vi "Main Data Log.vi"(8 "error in (no error)":errorcluster, 11 "main ref":T1) -> (0 "error out":errorcluster)   [LabVIEW 2025]
uses:
  controls/LAB-IQ UI Data.ctl
  <vilib>/Utility/file.llb/Write Delimited Spreadsheet (DBL).vi
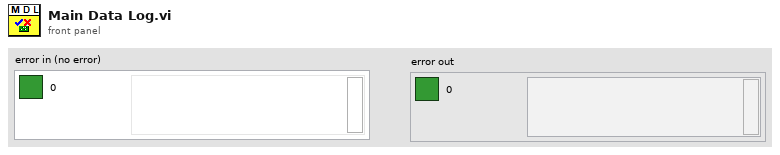
[diagram p1: front panel]
types:
  T1 = typedef "LAB-IQ UI Data.ctl" = cluster{"Main Home Screen":cluster{"GUI":refnum<vi>, "Platform Settings":refnum<vi>, "Configure":refnum<vi>, "Home":refnum<vi>, "EXIT":refnum<vi>, "service 2":refnum<vi>, "MainPage":refnum<vi>, "Analysis":refnum<vi>}, "Platform Settings":cluster{"mm/s  Surge":refnum<vi>, "Update Surge Speed":refnum<vi>, "Drive Error":refnum<vi>, "Disable Axis Jog Soft Limits":refnum<vi>, "mm/s  Sway":refnum<vi>, "Sway and Surge COM Status":refnum<vi>, "Heave COM Status":refnum<vi>, "Enable Platform":refnum<vi>, "Surge Forward Main":refnum<vi>, "Sway Right Main":refnum<vi>, "Sway Left Main":refnum<vi>, "Heave Down Main":refnum<vi>, "Heave Up main":refnum<vi>, "Update Sway Speed":refnum<vi>, "Update Heave Speed":refnum<vi>, "mm/s Heave":refnum<vi>, "mm/sec":refnum<vi>, "mm":refnum<vi>, "Surge Backward Main":refnum<vi>}, "Analysis Screen":cluster{"Analysis Home":refnum<vi>, "Surface Analysis":refnum<vi>, "Imaging":refnum<vi>, "Image Analysis":refnum<vi>, "Post Analysis":refnum<vi>}, "Config Screen":cluster{"Select Load Head":refnum<vi>, "Notes :":refnum<vi>, "FILE":refnum<vi>, "Sample ID :":refnum<vi>, "Operator ID :":refnum<vi>, "Operator Name :":refnum<vi>, "Auto":refnum<vi>}, "Motion Module":cluster{"zNL":refnum<vi>, "NL disp":refnum<vi>, "Rotary Tab":refnum<vi>, "Motion Direction:  3":refnum<vi>, "E.Velocity 2":refnum<vi>, "e.v/ssr 2":refnum<vi>, "Enter Fixed E.Velocity 2":refnum<vi>, "Enter Final SRR 2":refnum<vi>, "Enter initial SRR 2":refnum<vi>, "Enter Fixed SRR 2":refnum<vi>, "Enter the Final E.Velocity (m/s) 2":refnum<vi>, "Enter initial E.Velocity (m/s) 2":refnum<vi>, "Final Speed (RPM) 3":refnum<vi>, "Initial Speed (RPM) 2":refnum<vi>, "Enter the Final Velocity (m/s) 3":refnum<vi>, "Enter initial Velocity (m/s)  3":refnum<vi>, "Ramp Up 2":refnum<vi>, "TEST SELECTION":refnum<vi>, "SPEED SELECTION : ":refnum<vi>, "Angular Oscillation Set":refnum<vi>, "Traction":refnum<vi>, "Step Speed":refnum<vi>, "StepTable For Load-Speed":refnum<vi>, "StepTable For Speed":refnum<vi>, "Surge Forward MM":refnum<vi>, "Surge Backward MM":refnum<vi>, "M3 Image":refnum<vi>, "String 39":refnum<vi>, "Sway Left MM":refnum<vi>, "Sway Right MM":refnum<vi>, "Disable Axis Jog Soft Limits":refnum<vi>, "mm":refnum<vi>, "Heave Down MM":refnum<vi>, "Heave Up MM":refnum<vi>, "Wear Track Diameter (mm)":refnum<vi>, "Set WTD":refnum<vi>, "HomeScratch":refnum<vi>, "HomeRot":refnum<vi>, "PlaceModule":refnum<vi>, "Enter the Angle (Deg)":refnum<vi>, "Enter the Frequency (Hz)":refnum<vi>, "Motion Mode:":refnum<vi>, "LR Sway":refnum<vi>, "Rot Hor":refnum<vi>, "Scratch":refnum<vi>, "LR Cam":refnum<vi>, "MMBack":refnum<vi>, "MMNext":refnum<vi>, "Rot Ver":refnum<vi>, "Rotary Module Selection":refnum<vi>, "calculate rotary":refnum<vi>, "SPEED SELECTION : rotary":refnum<vi>, "Import 2":refnum<vi>, "Save 2":refnum<vi>, "File Path :  2":refnum<vi>, "String 45":refnum<vi>, "StepTable For Speed 3":refnum<vi>, "Enter the Speed(mm/sec)":refnum<vi>, "Enter the Speed(RPM)":refnum<vi>, "Enter Scratch Speed (mm/s):":refnum<vi>, "SwaySpeed Set":refnum<vi>, "Scartch Offset":refnum<vi>, "Motion type:":refnum<vi>, "HomeScratch 2":refnum<vi>, "Enter Scratch length (mm):":refnum<vi>, "Wear Track Diameter":refnum<vi>, "Rotary Speed Exced":refnum<vi>, "Scratch Mode":refnum<vi>, "No of Scratch":refnum<vi>}, "Environmental control":cluster{"Humidity  Status  3":refnum<vi>, "Low Temp  Status  2":refnum<vi>, "TK4 status 2":refnum<vi>, "Stage Temperature":refnum<vi>, "Sample Temperature":refnum<vi>, "Humidity (Amb)":refnum<vi>, "Clear List":refnum<vi>, "Add to list":refnum<vi>, "Wear":refnum<vi>, "Vibration":refnum<vi>, "Humidity (Chamber)":refnum<vi>, "Temperature (Chamber)":refnum<vi>, "ECR ":refnum<vi>, "Temperature (Amb)":refnum<vi>, "Microphone":refnum<vi>, "Acoustic Emission 3":refnum<vi>, "SNext":refnum<vi>, "APBack":refnum<vi>, "Enter the Temperature (°C):":refnum<vi>, "Enter the Stage \nTemperature (°C):":refnum<vi>, "Enter the Humidity (%Rh):":refnum<vi>, "Low Temp":refnum<vi>, "High Temp":refnum<vi>, "Humidity":refnum<vi>, "Sensors Picked":refnum<vi>}, "About Screen":cluster{"Password":refnum<vi>, "Home Service":refnum<vi>, "Advanced Setting":refnum<vi>, "About Tab":refnum<vi>, "ECR Port:":refnum<vi>, "Ramp Port:":refnum<vi>, "Installation/Replacement completed":refnum<vi>, "Loahead":refnum<vi>, "Heave and Surge COM Port:":refnum<vi>, "Sway COM Port:":refnum<vi>, "Temp Modbus:":refnum<vi>, "Humidity Port:":refnum<vi>, "Edit Gain Constants":refnum<vi>, "Save Gain Constants":refnum<vi>}, "Main Screen":cluster{"Main Screen Tab":refnum<vi>, "Angle and Frequency":refnum<vi>, "Stroke (mm)":refnum<vi>, "Angle (Deg)":refnum<vi>, "Main Speed Tab":refnum<vi>, "MTM MOTOR DISPLAY":refnum<vi>, "Disc Speed (m/sec)":refnum<vi>, "Ball Speed (m/sec)":refnum<vi>, "Disc Speed (RPM)":refnum<vi>, "Ball Speed (RPM)":refnum<vi>, "SPEED TAB":refnum<vi>, "Speed (m/sec)":refnum<vi>, "Set Speed (m/sec)":refnum<vi>, "Speed (RPM)":refnum<vi>, "Set Speed":refnum<vi>, "Time Tab":refnum<vi>, "Time ( HH:MM:SS ) 2":refnum<vi>, "Test Duration":refnum<vi>, "Test Duration 4":refnum<vi>, "TEST CYCLE":refnum<vi>, "TOTAL CYCLES":refnum<vi>, "Set Load (N)":refnum<vi>, "Temp Tabs":refnum<vi>, "Heater":refnum<vi>, "TK4 status":refnum<vi>, "ChamberTemp":refnum<vi>, "SetTmp":refnum<vi>, "Controller  Status":refnum<vi>, "ChamberTemp 2":refnum<vi>, "SetTmp 2":refnum<vi>, "Controller  Status 2":refnum<vi>, "ChamberTemp 3":refnum<vi>, "SetTmp 3":refnum<vi>, "Cooling":refnum<vi>, "Load Communication":refnum<vi>, "Ambient \nTemperature":refnum<vi>, "HumCOMStatus":refnum<vi>, "Ambient\n Humidity":refnum<vi>, "Freq (Hz)":refnum<vi>, "Load En":refnum<vi>, "NLt":refnum<vi>, "zNL 2":refnum<vi>, "Humidity On":refnum<vi>, "humidity disp":refnum<vi>, "Set Humidity":refnum<vi>, "NL disp 2":refnum<vi>, "Humidity On 2":refnum<vi>, "humidity disp 2":refnum<vi>, "Set Humidity 2":refnum<vi>, "NL disp 3":refnum<vi>, "AppLoadSeq scratch":refnum<vi>, "Stop Scratch":refnum<vi>, "ClrLog":refnum<vi>, "Trip Log":refnum<vi>, "STOP":refnum<vi>, "Start Test":refnum<vi>, "Test status":refnum<vi>, "AR Led":refnum<vi>, "Data":refnum<vi>, "Health":refnum<vi>, "Sway COM Status":refnum<vi>, "Heave COM Status":refnum<vi>, "Grp Tab":refnum<vi>, "Sub Graph":refnum<vi>, "SD (mm)":refnum<vi>, "Siliding distance Reset Graph":refnum<vi>, "SDGp":refnum<vi>, "Humidity Reset Graph":refnum<vi>, "HumrGp":refnum<vi>, "Acoustic Emission (mV)":refnum<vi>, "Aqucostic Reset Graph":refnum<vi>, "gACQUOS":refnum<vi>, "ECR RESET":refnum<vi>, "ECR":refnum<vi>, "Temperature Reset":refnum<vi>, "Acoustic Emission (mV) 2":refnum<vi>, "Aqucostic Reset Graph 2":refnum<vi>, "gACQUOS 2":refnum<vi>, "ECR RESET 2":refnum<vi>, "ECR 2":refnum<vi>, "Temperature Reset 2":refnum<vi>, "Temperature (deg c)":refnum<vi>, "Speed Reset Graph":refnum<vi>, "Speed Tab":refnum<vi>, "MTM DISC  SPEED":refnum<vi>, "MTM BALL SPEED":refnum<vi>, "speed mm/sec":refnum<vi>, "Hymidity":refnum<vi>, "Humidity Disable trip":refnum<vi>, "CoF Trip  2":refnum<vi>, "Depth Trip":refnum<vi>, "Weart Deapth":refnum<vi>, "Depth Reset Graph":refnum<vi>, "Weart":refnum<vi>, "Depthz":refnum<vi>, "Depth (µm)":refnum<vi>, "WearGp":refnum<vi>, "NL Trip 2":refnum<vi>, "Load pid":refnum<vi>, "Load Disable Trip":refnum<vi>, "Load Reset Graph":refnum<vi>, "NL Display 4":refnum<vi>, "Main Chart 3":refnum<vi>, "BACK":refnum<vi>, "Depth Trip 2":refnum<vi>, "COF TRIP ":refnum<vi>, "Friction Force (N)":refnum<vi>, "FF Reset Graph":refnum<vi>, "FF Disable Trip":refnum<vi>, "FF TRIP":refnum<vi>, "COF Disable Trip":refnum<vi>, "COF Reset Graph":refnum<vi>, "Start Test Temp":refnum<vi>, "zFF":refnum<vi>, "Friction Force (N) Graph":refnum<vi>, "Coefficient of Friction":refnum<vi>, "Scratch Start Test":refnum<vi>, "FF Tab":refnum<vi>, "Cyclic Friction Force (N)":refnum<vi>, "CZ FF":refnum<vi>, "Cyclic Friction Force (N) Graph":refnum<vi>, "Cyclic Coefficient of Friction":refnum<vi>, "Cyclic FF TRIP":refnum<vi>, "Cyclic FF Disable Trip":refnum<vi>, "cyclic COF Disable Trip":refnum<vi>, "cyclic COF TRIP":refnum<vi>, "cyclic COF Reset Graph":refnum<vi>, "Cyclic FF Reset Graph":refnum<vi>, "Test Trip":refnum<vi>, "Multi Scratch Pass":refnum<vi>}, "Loading":cluster{"Indentation":refnum<vi>, "Reference Sample":refnum<vi>, "Load Cell Communication Slide":refnum<vi>, "com 3":refnum<vi>, "com":refnum<vi>, "DecaForce COM Status":refnum<vi>, "Update":refnum<vi>, "Clear 3":refnum<vi>, "seq":refnum<vi>, "Stribeck table":refnum<vi>, "Stribeck Table  For loading":refnum<vi>, "Loading Mode":refnum<vi>, "Enter the Final Load (N)":refnum<vi>, "Enter the CoF Trip":refnum<vi>, "Enter the Friction Force Trip":refnum<vi>, "Enter the Normal load Trip":refnum<vi>, "Enter the Load  (N)":refnum<vi>, "KiloForce":refnum<vi>, "DecaForce ":refnum<vi>, "MicroForce":refnum<vi>, "LHBack":refnum<vi>, "LHNext":refnum<vi>, "Enter the Loading Rate (N/min)":refnum<vi>, "Message":refnum<vi>, "Warning 2":refnum<vi>, "SSP 0.75":refnum<vi>, "SSP 0.5":refnum<vi>, "SSP 0.3":refnum<vi>, "Warning":refnum<vi>, "gui GIF":refnum<vi>, "Communication is established":refnum<vi>, "AppLoad 4":refnum<vi>, "Multipoint":refnum<vi>, "Load Selection":refnum<vi>}, "PID":cluster{"Ramp MulFac":refnum<vi>, "pulses LoadDiffRamp(2..10)":refnum<vi>, "PulseControlRamp(diff<=3N)":refnum<vi>, "SetLoadDeadband(%) Load(0-10N)":refnum<vi>, "PID gains out delay (microForce)":refnum<vi>, "Ramp":refnum<vi>, "Gain 2":refnum<vi>, "pulses LoadDiff(2..10)":refnum<vi>, "pulses LoadDiff(11..50)":refnum<vi>, "PulseControl(diff<=3N)":refnum<vi>, "SetLoadDeadband(%)  2":refnum<vi>, "Dummy Run":refnum<vi>, "Vertical load (N)":refnum<vi>, "AutoTune":refnum<vi>, "Offset 3 ":refnum<vi>, "apply load":refnum<vi>, "Offset  3":refnum<vi>, "apply load 2":refnum<vi>, "Enter ByPass Load":refnum<vi>, "reinit 3":refnum<vi>, "output range delay":refnum<vi>, "PID gains out delay":refnum<vi>, "Bypass Load":refnum<vi>, "pulsesSent":refnum<vi>, "pulses ":refnum<vi>, "actpid":refnum<vi>, "gFF Rot":refnum<vi>, "pulses LoadDiff(21..1000)":refnum<vi>, "Delay":refnum<vi>, "deadband":refnum<vi>}, "Config Parameters":cluster{"Tab Control 3":refnum<vi>, "Tab Control 19":refnum<vi>, "SAMPLES":refnum<vi>, "Re-initilaize":refnum<vi>, "Filter ON/OFF":refnum<vi>, "TracHomeSurgeOffsetCounts 10MM":refnum<vi>, "TracHomeSwayOffsetCounts 10MM":refnum<vi>, "Acoustic Emission:":refnum<vi>, "Apply Filter (FF)":refnum<vi>, "Filter% 2":refnum<vi>, "Apply Filter (Load)":refnum<vi>, "Filter% ":refnum<vi>, "Sway distance (mm)":refnum<vi>, "Surge distance (mm)":refnum<vi>, "DataSavingLoopDelay(ms)":refnum<vi>, "SAVE 2":refnum<vi>, "Enter Distance":refnum<vi>, "Sway Counts:":refnum<vi>, "Distance (mm): 3":refnum<vi>, "Surge Counts:":refnum<vi>, "Distance (mm): 2":refnum<vi>, "Distance (mm):":refnum<vi>, "Heave Counts:":refnum<vi>, "LRMHomeSurgeOffsetCounts":refnum<vi>, "LRMHomeSwayOffsetCounts":refnum<vi>, "TracHomeSurgeOffsetCounts 20MM":refnum<vi>, "TracHomeSwayOffsetCounts 20MM":refnum<vi>, "RotHomeSwayOffsetCounts":refnum<vi>, "RotHomeSurgeOffsetCounts":refnum<vi>, "Heave distance":refnum<vi>, "Zmm":refnum<vi>, "Heave Pulses/mm":refnum<vi>, "Surge Pulses/mm":refnum<vi>, "Sway Pulses/mm":refnum<vi>, "Heave Pitch":refnum<vi>, "Surge Pitch":refnum<vi>, "Sway Pitch":refnum<vi>, "Heave PPR":refnum<vi>, "Surge PPR":refnum<vi>, "Sway PPR":refnum<vi>, "Tab Control 5":refnum<vi>, "Tab Control 14":refnum<vi>, "Tab Control 26":refnum<vi>, "AE":refnum<vi>, "Heave Loop Delay":refnum<vi>, "Heave PID Speed":refnum<vi>, "Surge Jog Speed":refnum<vi>, "Heave Jog Speed":refnum<vi>, "Sway Loop Delay":refnum<vi>, "Sway PID Speed":refnum<vi>, "Sway Jog Speed":refnum<vi>}, "Loading Com Port":cluster{"ClearAll":refnum<vi>, "Mz(Nm)":refnum<vi>, "My(Nm)":refnum<vi>, "Mx(Nm)":refnum<vi>, "Save Dwell":refnum<vi>, "Mx ":refnum<vi>, "My ":refnum<vi>, "Mz":refnum<vi>, "Fx(N)":refnum<vi>, "Fy(N)":refnum<vi>, "Fz(N)":refnum<vi>, "ZeroAll":refnum<vi>, "Acq Delay (ms)":refnum<vi>, "Burst Delay (ms)":refnum<vi>, "model":refnum<vi>, "SN":refnum<vi>, "FFx(N)":refnum<vi>, "Sensor IP":refnum<vi>, "Port":refnum<vi>, "FFy(N)":refnum<vi>, "Load(N)":refnum<vi>, "delete Handle":refnum<vi>, "Create Handle":refnum<vi>, "ft_data":refnum<vi>, "ft_range":refnum<vi>, "ft_data 2":refnum<vi>, "stop 6":refnum<vi>, "running_flag":refnum<vi>, "ft_udp_handle":refnum<vi>, "get-data-return":refnum<vi>, "get-range-return":refnum<vi>, "zero-return":refnum<vi>, "filter-return":refnum<vi>, "initial-return":refnum<vi>, "deleteHandle-result":refnum<vi>, "Load Cell Temp":refnum<vi>}, "Heave AND Surge":cluster{"SURGE POSE":refnum<vi>, "error out Read":refnum<vi>, "HEAVE POSE":refnum<vi>, "State":refnum<vi>, "Homed":refnum<vi>, "Sequence ID":refnum<vi>, "error out Write":refnum<vi>, "faultCode":refnum<vi>, "Ack ID":refnum<vi>, "SPEED":refnum<vi>, "Distance":refnum<vi>, "Mode Command":refnum<vi>, "Heave and Surge Read":refnum<vi>, "Read Heave Temp":refnum<vi>, "Spare 15":refnum<vi>, "Spare 14":refnum<vi>, "Spare 13":refnum<vi>, "Spare 12":refnum<vi>, "Spare 11":refnum<vi>, "Spare 10":refnum<vi>, "Spare 9":refnum<vi>, "Spare 8":refnum<vi>, "Spare 7":refnum<vi>, "Spare 6":refnum<vi>, "Spare 5":refnum<vi>, "Spare 4":refnum<vi>, "Spare 2":refnum<vi>, "Spare 1":refnum<vi>, "Node Id":refnum<vi>, "Spare 3":refnum<vi>, "SPARE 4":refnum<vi>, "SPARE 3":refnum<vi>, "SPARE 2":refnum<vi>, "SPARE 1":refnum<vi>, "fwMajor":refnum<vi>, "fwMinor":refnum<vi>, "Manual Write":refnum<vi>, "Heave and Surge Write":refnum<vi>}, "New PID LOGIC":cluster{"Fine Tune Zone":refnum<vi>, "PID SDelay":refnum<vi>, "Max_pos_limit":refnum<vi>, "Min_pos_limit":refnum<vi>, "i_limit":refnum<vi>, "pct_scale":refnum<vi>, "Deadband":refnum<vi>, "Kd":refnum<vi>, "Ki":refnum<vi>, "Kp":refnum<vi>, "Current Position":refnum<vi>, "Set Load":refnum<vi>, "Current Load":refnum<vi>, "Pulse delta":refnum<vi>, "Init Step":refnum<vi>, "Max Step Linit":refnum<vi>}, "SWAY ":cluster{"fwMajor":refnum<vi>, "Homed":refnum<vi>, "Rotary POSE":refnum<vi>, "State":refnum<vi>, "SWAY POSE":refnum<vi>, "Ack ID":refnum<vi>, "faultCode":refnum<vi>, "Node Id":refnum<vi>, "fwMinor":refnum<vi>, "Spare 6":refnum<vi>, "Spare 5":refnum<vi>, "Spare 4":refnum<vi>, "Spare 3":refnum<vi>, "Spare 2":refnum<vi>, "Spare 1":refnum<vi>, "Spare 7":refnum<vi>, "SPARE  5":refnum<vi>, "error out Write  SWAY ":refnum<vi>, "error out Read SWAY ":refnum<vi>, "Manual Write SWAY ":refnum<vi>, "SWAY WRITE":refnum<vi>, "SPARE  4":refnum<vi>, "SPARE  3":refnum<vi>, "SPARE 2":refnum<vi>, "SPARE 1":refnum<vi>, "Spare 15":refnum<vi>, "Spare 14":refnum<vi>, "Spare 13":refnum<vi>, "Spare 12":refnum<vi>, "Spare 11":refnum<vi>, "Spare 9":refnum<vi>, "Spare 8":refnum<vi>, "SPEED":refnum<vi>, "Distance":refnum<vi>, "Mode Command":refnum<vi>, "Sequence ID":refnum<vi>, "SWAY READ":refnum<vi>, "Spare 10":refnum<vi>, "Read SWAY Temp":refnum<vi>}, "Analysis Screen":cluster{"Analysis Home":refnum<vi>, "Refresh 2":refnum<vi>, "MEAN 4":refnum<vi>, "SD 4":refnum<vi>, "VARIANCE 4":refnum<vi>, "MEAN  3":refnum<vi>, "SD  3":refnum<vi>, "VARIANCE  3":refnum<vi>, "MEAN 2":refnum<vi>, "SD  2":refnum<vi>, "VARIANCE 2":refnum<vi>, "MEAN":refnum<vi>, "SD":refnum<vi>, "VARIANCE":refnum<vi>, "File 4 Discription":refnum<vi>, "OPEN 4":refnum<vi>, "File Name 4":refnum<vi>, "OPEN 3":refnum<vi>, "File 3 Discription":refnum<vi>, "File Name 3":refnum<vi>, "Y-AXIS":refnum<vi>, "X-AXIS":refnum<vi>, "XY Graph":refnum<vi>, "File Name 2":refnum<vi>, "File Name 1":refnum<vi>, "OPEN 2":refnum<vi>, "OPEN 1":refnum<vi>, "File 1 Discription ":refnum<vi>, "File 2 Discription":refnum<vi>}}
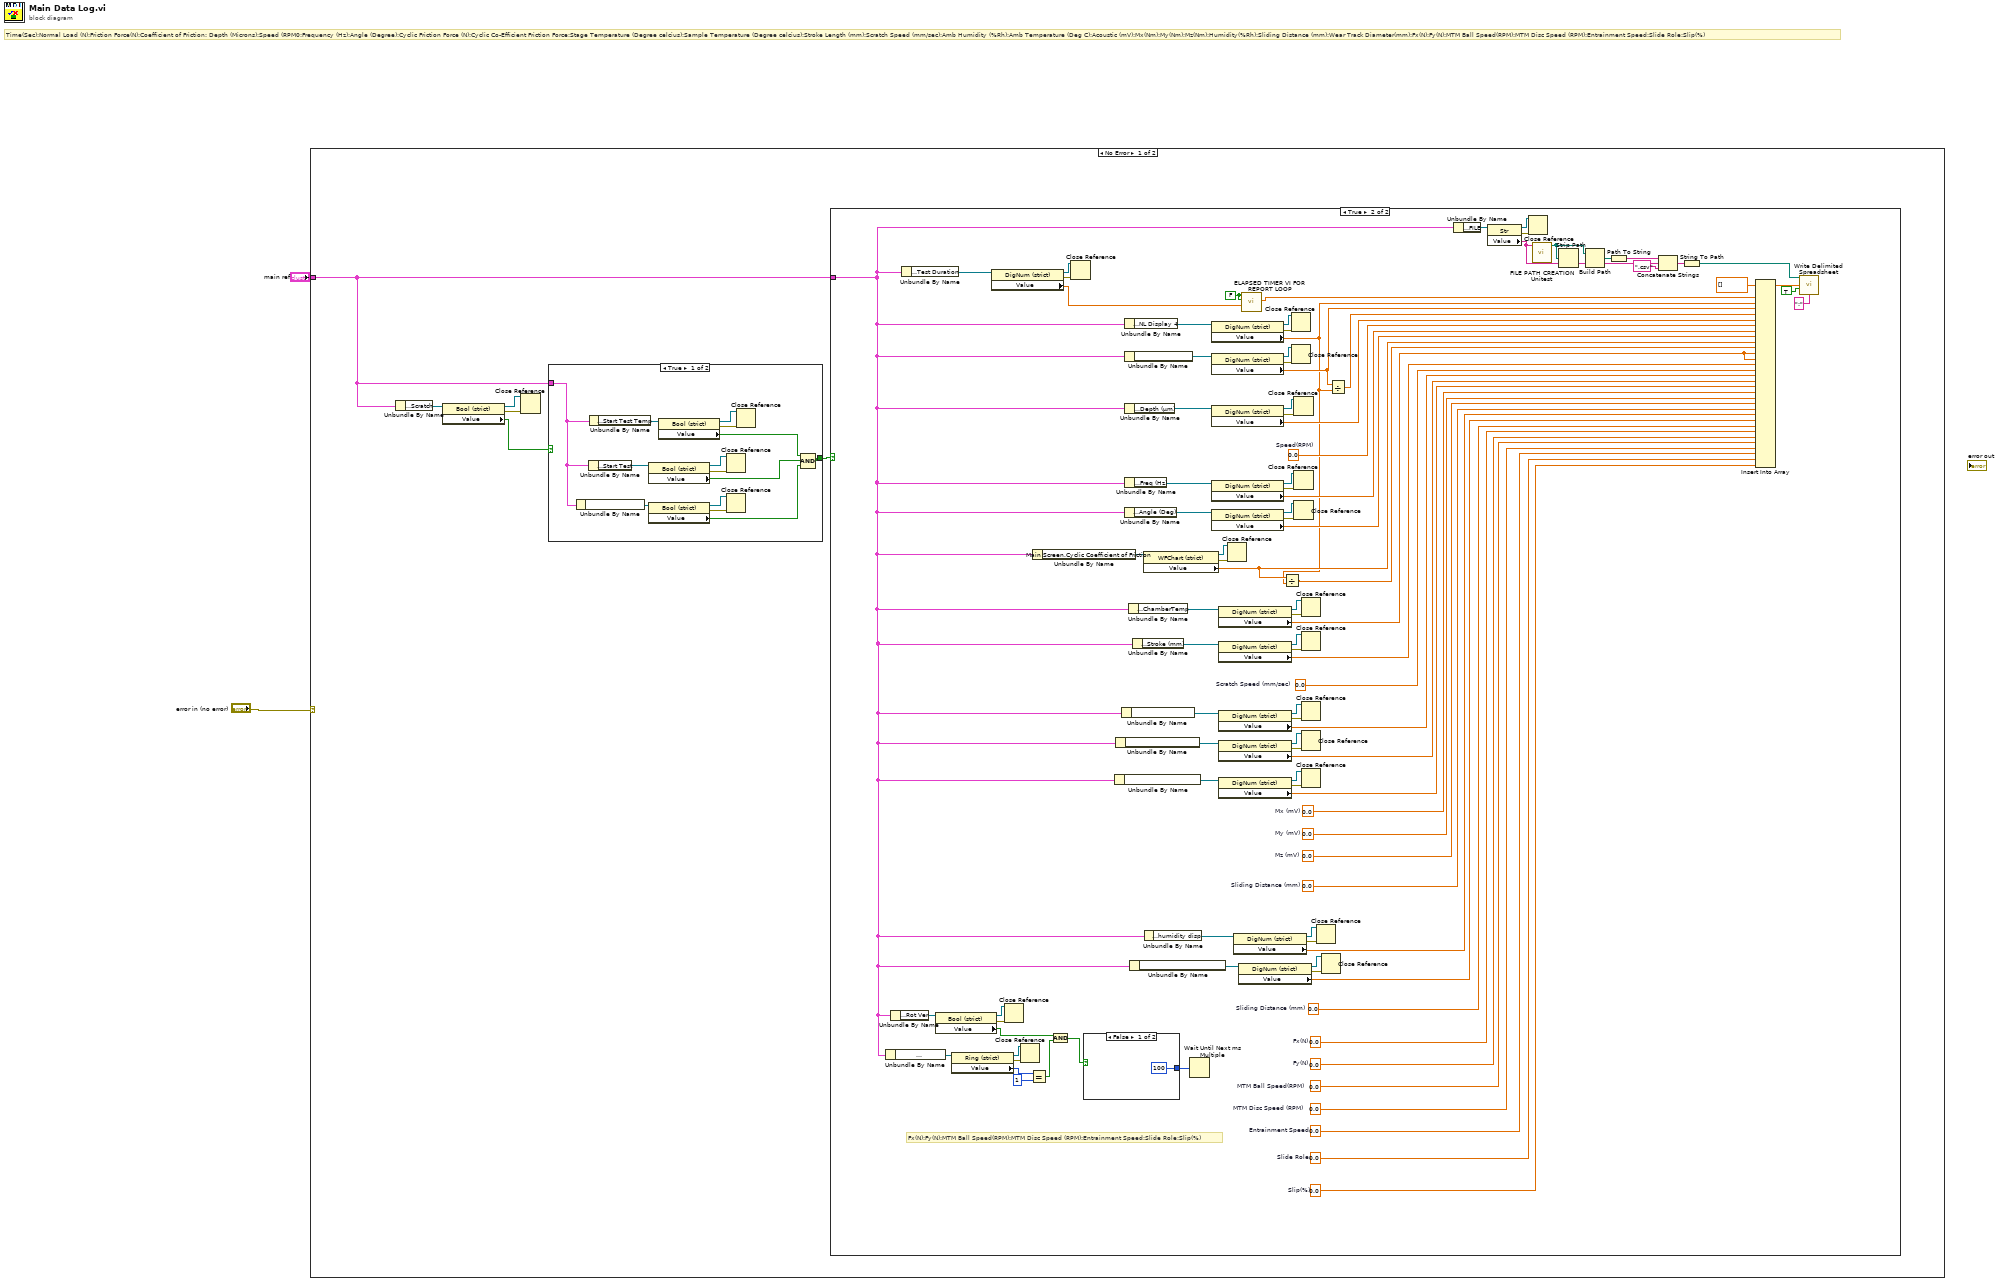
[diagram p0: block diagram]
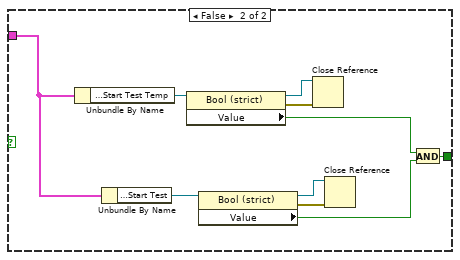
[diagram p2: hidden frame]
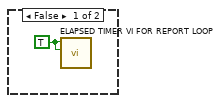
[diagram p3: hidden frame]
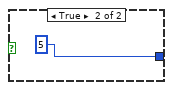
[diagram p4: hidden frame]
diagram:
  # "Time(Sec):Normal Load (N):Friction Force(N):Coefficient of Friction: Depth (Microns):Speed (RPM0:Frequency (Hz):Angle (Degree):Cyclic Friction Force (N):Cyclic Co-Efficient Friction Force:Stage Temperature (Degree celcius):Sample Temperature (Degree celcius):Stroke Length (mm):Scratch Speed (mm/sec):Amb Humidity (%Rh):Amb Temperature (Deg C):Acoustic (mV):Mx(Nm):My(Nm);Mz(Nm):Humidity(%Rh):Sliding Distance (mm):Wear Track Diameter(mm):Fx(N):Fy(N):MTM Ball Speed(RPM):MTM Disc Speed (RPM):Entrainment Speed:Slide Role:Slip(%)"
  n1 = case shown="No Error" "error in (no error)" {
    tunnel: "main ref" -> [w4 _]
    frame No Error {
      n2 = Unbundle By Name(w4) -> ("Motion Module.Scratch"=w7:refnum<vi>)
      n3 = property class="Bool (strict)"(reference=w7) -> (reference out=w8:refnum<vi>, error out=w6:errorcluster, "Value"=w5:bool)  [unwired: 1 in]
      n4 = Close Reference(reference=w8, error in (no error)=w6) -> ()  [unwired: 1 out]
      n5 = case shown="True" w5 {
        tunnel: w4 -> [w10 w26]
        tunnel: [w14 w23] -> w3
        frame True {
          n6 = Unbundle By Name(w10) -> ("Main Screen.Scratch Start Test"=w12:refnum<vi>)
          n7 = Unbundle By Name(w10) -> ("Main Screen.Start Test"=w18:refnum<vi>)
          n8 = Unbundle By Name(w10) -> ("Main Screen.Start Test Temp"=w21:refnum<vi>)
          n9 = property class="Bool (strict)"(reference=w18) -> (reference out=w17:refnum<vi>, error out=w19:errorcluster, "Value"=w15:bool)  [unwired: 1 in]
          n10 = property class="Bool (strict)"(reference=w12) -> (reference out=w13:refnum<vi>, error out=w11:errorcluster, "Value"=w9:bool)  [unwired: 1 in]
          n11 = property class="Bool (strict)"(reference=w21) -> (reference out=w22:refnum<vi>, error out=w20:errorcluster, "Value"=w16:bool)  [unwired: 1 in]
          n12 = Close Reference(reference=w17, error in (no error)=w19) -> ()  [unwired: 1 out]
          n13 = Close Reference(reference=w13, error in (no error)=w11) -> ()  [unwired: 1 out]
          n14 = Close Reference(reference=w22, error in (no error)=w20) -> ()  [unwired: 1 out]
          n15 = Compound Arithmetic op=AND(w16, w15, w9) -> (w14:bool)
        }
        frame False {
          n16 = Unbundle By Name(w26) -> ("Main Screen.Start Test Temp"=w31:refnum<vi>)
          n17 = Unbundle By Name(w26) -> ("Main Screen.Start Test"=w28:refnum<vi>)
          n18 = property class="Bool (strict)"(reference=w31) -> (reference out=w32:refnum<vi>, error out=w30:errorcluster, "Value"=w25:bool)  [unwired: 1 in]
          n19 = property class="Bool (strict)"(reference=w28) -> (reference out=w27:refnum<vi>, error out=w29:errorcluster, "Value"=w24:bool)  [unwired: 1 in]
          n20 = Close Reference(reference=w32, error in (no error)=w30) -> ()  [unwired: 1 out]
          n21 = Close Reference(reference=w27, error in (no error)=w29) -> ()  [unwired: 1 out]
          n22 = And(x=w25, y=w24) -> (x .and. y?=w23:bool)
        }
      }
      n23 = case shown="True" w3 {
        tunnel: w4 -> [_ w36]
        frame False {
          w33 = TRUE ("PAUSE")
          n24 = call "ELAPSED TIMER VI FOR REPORT LOOP.vi"("RESET"=w33, "PAUSE"=w33) -> ()  [unwired: 7 in, 3 out]
        }
        frame True {
          w58 = 0.0  # Slip(%)
          w59 = 0.0  # Slide Role:
          w60 = 0.0  # Entrainment Speed
          w61 = 0.0  # MTM Disc Speed (RPM)
          w62 = 0.0  # MTM Ball Speed(RPM)
          w63 = 0.0  # Fy(N)
          w64 = 0.0  # Fx(N)
          w69 = 0.0  # Mz (mV)
          w70 = 0.0  # My (mV)
          w71 = 0.0  # Mx (mV)
          w65 = 0.0  # Sliding Distance (mm)
          w68 = 0.0  # Sliding Distance (mm)
          w76 = 0.0  # Scratch Speed (mm/sec)
          w99 = 0.0  # Speed(RPM)
          w126 = FALSE ("PAUSE")
          # "Fx(N):Fy(N):MTM Ball Speed(RPM):MTM Disc Speed (RPM):Entrainment Speed:Slide Role:Slip(%)"
          n25 = Unbundle By Name(w36) -> ("Motion Module.Motion Mode:"=w41:refnum<vi>)
          n26 = Unbundle By Name(w36) -> ("Motion Module.Rot Ver"=w46:refnum<vi>)
          n27 = Unbundle By Name(w36) -> ("Main Screen.Test Duration"=w54:refnum<vi>)
          n28 = property class="Bool (strict)"(reference=w46) -> (reference out=w44:refnum<vi>, error out=w45:errorcluster, "Value"=w38:bool)  [unwired: 1 in]
          n29 = property class="Ring (strict)"(reference=w41) -> (reference out=w43:refnum<vi>, error out=w42:errorcluster, "Value"=w40:u16)  [unwired: 1 in]
          n30 = property class="DigNum (strict)"(reference=w54) -> (reference out=w55:refnum<vi>, error out=w56:errorcluster, "Value"=w53:dbl)  [unwired: 1 in]
          n31 = Close Reference(reference=w44, error in (no error)=w45) -> ()  [unwired: 1 out]
          n32 = Close Reference(reference=w43, error in (no error)=w42) -> ()  [unwired: 1 out]
          n33 = Equal?(x=w40, y=u16 1) -> (x = y?=w37:bool)
          n34 = Unbundle By Name(w36) -> ("Main Screen.Cyclic Coefficient of Friction"=w52:refnum<vi>)
          n35 = And(x=w38, y=w37) -> (x .and. y?=w35:bool)
          n36 = Close Reference(reference=w55, error in (no error)=w56) -> ()  [unwired: 1 out]
          n37 = case shown="False" w35 {
            tunnel: [u32 100 ("millisecond multiple") u32 5 ("millisecond multiple")] -> w34
            frame False {
            }
            frame True {
            }
          }
          n38 = Unbundle By Name(w36) -> ("Main Screen.Acoustic Emission (mV)"=w80:refnum<vi>)
          n39 = Unbundle By Name(w36) -> ("Main Screen.Ambient \nTemperature"=w86:refnum<vi>)
          n40 = Unbundle By Name(w36) -> ("Main Screen.Ambient\n Humidity"=w89:refnum<vi>)
          n41 = Unbundle By Name(w36) -> ("Main Screen.NL Display 4"=w120:refnum<vi>)
          n42 = Unbundle By Name(w36) -> ("Main Screen.Friction Force (N)"=w114:refnum<vi>)
          n43 = Unbundle By Name(w36) -> ("Main Screen.Depth (µm)"=w111:refnum<vi>)
          n44 = Unbundle By Name(w36) -> ("Main Screen.Freq (Hz)"=w105:refnum<vi>)
          n45 = Unbundle By Name(w36) -> ("Main Screen.Angle (Deg)"=w104:refnum<vi>)
          n46 = Unbundle By Name(w36) -> ("Main Screen.ChamberTemp"=w100:refnum<vi>)
          n47 = Unbundle By Name(w36) -> ("Motion Module.Wear Track Diameter (mm)"=w83:refnum<vi>)
          n48 = Unbundle By Name(w36) -> ("Main Screen.Stroke (mm)"=w93:refnum<vi>)
          n49 = property class="WFChart (strict)"(reference=w52) -> (reference out=w47:refnum<vi>, error out=w51:errorcluster, "Value"=w50:dbl)  [unwired: 1 in]
          n50 = Unbundle By Name(w36) -> ("Main Screen.humidity disp"=w79:refnum<vi>)
          n51 = Wait Until Next ms Multiple(millisecond multiple=w34) -> ()  [unwired: 1 out]
          n52 = property class="DigNum (strict)"(reference=w120) -> (reference out=w119:refnum<vi>, error out=w118:errorcluster, "Value"=w49:dbl)  [unwired: 1 in]
          n53 = property class="DigNum (strict)"(reference=w114) -> (reference out=w115:refnum<vi>, error out=w116:errorcluster, "Value"=w113:dbl)  [unwired: 1 in]
          n54 = property class="DigNum (strict)"(reference=w111) -> (reference out=w109:refnum<vi>, error out=w110:errorcluster, "Value"=w108:dbl)  [unwired: 1 in]
          n55 = property class="DigNum (strict)"(reference=w105) -> (reference out=w107:refnum<vi>, error out=w106:errorcluster, "Value"=w98:dbl)  [unwired: 1 in]
          n56 = property class="DigNum (strict)"(reference=w104) -> (reference out=w102:refnum<vi>, error out=w103:errorcluster, "Value"=w97:dbl)  [unwired: 1 in]
          n57 = property class="DigNum (strict)"(reference=w100) -> (reference out=w96:refnum<vi>, error out=w101:errorcluster, "Value"=w95:dbl)  [unwired: 1 in]
          n58 = property class="DigNum (strict)"(reference=w93) -> (reference out=w94:refnum<vi>, error out=w92:errorcluster, "Value"=w91:dbl)  [unwired: 1 in]
          n59 = property class="DigNum (strict)"(reference=w89) -> (reference out=w88:refnum<vi>, error out=w90:errorcluster, "Value"=w75:dbl)  [unwired: 1 in]
          n60 = property class="DigNum (strict)"(reference=w86) -> (reference out=w87:refnum<vi>, error out=w85:errorcluster, "Value"=w74:dbl)  [unwired: 1 in]
          n61 = property class="DigNum (strict)"(reference=w80) -> (reference out=w73:refnum<vi>, error out=w81:errorcluster, "Value"=w72:dbl)  [unwired: 1 in]
          n62 = Close Reference(reference=w47, error in (no error)=w51) -> ()  [unwired: 1 out]
          n63 = property class="DigNum (strict)"(reference=w79) -> (reference out=w77:refnum<vi>, error out=w78:errorcluster, "Value"=w67:dbl)  [unwired: 1 in]
          n64 = property class="DigNum (strict)"(reference=w83) -> (reference out=w82:refnum<vi>, error out=w84:errorcluster, "Value"=w66:dbl)  [unwired: 1 in]
          n65 = call "ELAPSED TIMER VI FOR REPORT LOOP.vi"("TARGET"=w53, "RESET"=w126, "PAUSE"=w126) -> ("ELAPSED TIMER"=w125:dbl)  [unwired: 6 in, 2 out]
          n66 = Divide(x=w50, y=w49) -> (x/y=w48:dbl)
          n67 = Close Reference(reference=w119, error in (no error)=w118) -> ()  [unwired: 1 out]
          n68 = Close Reference(reference=w115, error in (no error)=w116) -> ()  [unwired: 1 out]
          n69 = Close Reference(reference=w109, error in (no error)=w110) -> ()  [unwired: 1 out]
          n70 = Close Reference(reference=w107, error in (no error)=w106) -> ()  [unwired: 1 out]
          n71 = Close Reference(reference=w102, error in (no error)=w103) -> ()  [unwired: 1 out]
          n72 = Close Reference(reference=w96, error in (no error)=w101) -> ()  [unwired: 1 out]
          n73 = Close Reference(reference=w94, error in (no error)=w92) -> ()  [unwired: 1 out]
          n74 = Close Reference(reference=w88, error in (no error)=w90) -> ()  [unwired: 1 out]
          n75 = Close Reference(reference=w87, error in (no error)=w85) -> ()  [unwired: 1 out]
          n76 = Close Reference(reference=w73, error in (no error)=w81) -> ()  [unwired: 1 out]
          n77 = Close Reference(reference=w77, error in (no error)=w78) -> ()  [unwired: 1 out]
          n78 = Close Reference(reference=w82, error in (no error)=w84) -> ()  [unwired: 1 out]
          n79 = Divide(x=w113, y=w49) -> (x/y=w112:dbl)
          n80 = Unbundle By Name(w36) -> ("Config Screen.FILE"=w127:refnum<vi>)
          n81 = property class="Str"(reference=w127) -> (reference out=w129:refnum<vi>, error out=w128:errorcluster, "Value"=w57:string)  [unwired: 1 in]
          n82 = Close Reference(reference=w129, error in (no error)=w128) -> ()  [unwired: 1 out]
          n83 = call "FILE PATH CREATION Unitest.vi"("FILE NAME :"=w57) -> ("FILE OUT"=w130:path)  [unwired: 9 in, 1 out]
          n84 = Strip Path(path=w130) -> (name=w133:string)  [unwired: 1 out]
          n85 = Build Path(base path=w130, name or relative path=w133) -> (appended path=w134:path)
          n86 = Path To String(path=w134) -> (string=w131:string)
          n87 = Concatenate Strings(w131, w57, ".csv" ("string")) -> (w132:string)
          n88 = String To Path(string=w132) -> (path=w117:path)
          n89 = Insert Into Array(array=dbl[] [], new element #1=w125, new element #2=w49, new element #3=w113, new element #4=w112, new element #5=w108, new element #6=w99, new element #7=w98, new element #8=w97, new element #9=w50, new element #10=w48, new element #11=w95, new element #12=w95, new element #13=w91, new element #14=w76, new element #15=w75, new element #16=w74, new element #17=w72, new element #18=w71, new element #19=w70, new element #20=w69, new element #21=w68, new element #22=w67, new element #23=w66, new element #24=w65, new element #25=w64, new element #26=w63, new element #27=w62, new element #28=w61, new element #29=w60, new element #30=w59, new element #31=w58) -> (w121:dbl[])  [unwired: 1 in]
          n90 = call-poly <vilib>:"Write Delimited Spreadsheet.vi"("file path (dialog if empty)"=w117, "1D data"=w121, "append to file? (new file:F)"=TRUE, "delimiter (\\t)"=":" ("delimiter (Tab)")) -> ()  [unwired: 10 in, 2 out]
        }
      }
    }
    frame Error {
    }
  }
